vi "PPS Close.vi"(8 "error in (no error)":errorcluster, 11 "IT-M3904D in":refnum<class "IT-M3904D.lvclass">) -> (0 "error out":errorcluster, 3 "IT-M3904D out":refnum<class "IT-M3904D.lvclass">)   [LabVIEW 2023, in "HardwareAbstractionLayer_LVOOP.lvlib" / "IT-M3904D.lvclass"]
uses:
  IT-M3904D.lvclass
  <instrlib>/IT-M3900D/IT-M3900D.lvlib
  PowerSupply.lvclass
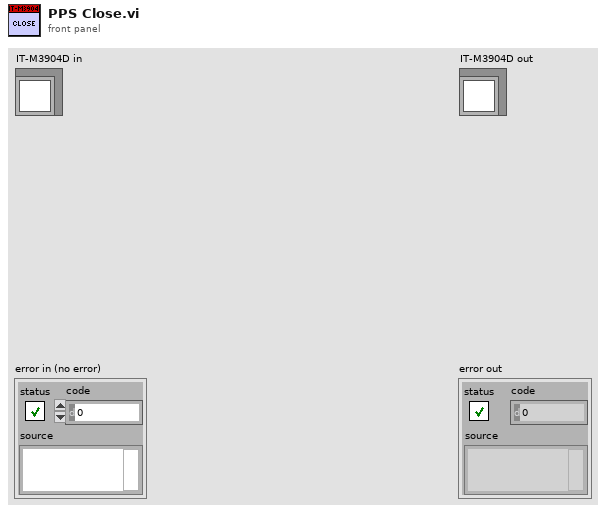
[diagram p1: front panel]
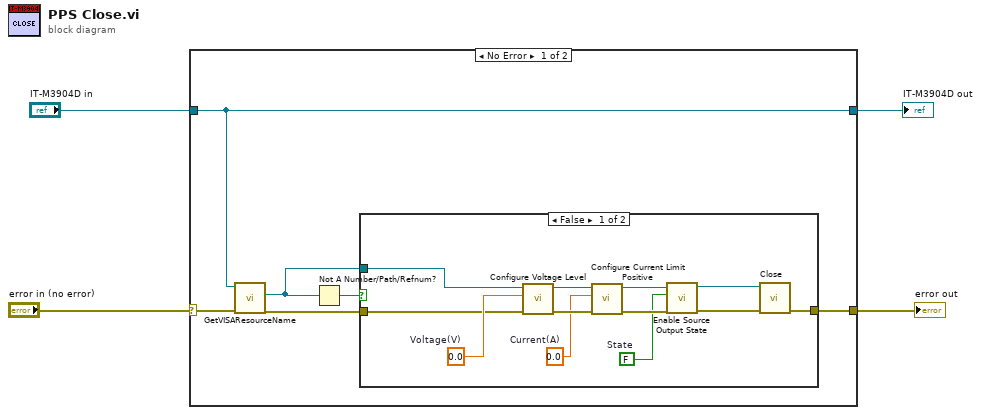
[diagram p0: block diagram]
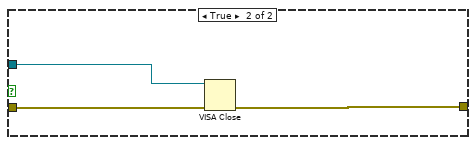
[diagram p2: hidden frame]
diagram:
  n1 = case shown="No Error" "error in (no error)" {
    selector: "error in (no error)" -> [w9 w26]
    tunnel: [w10 w26] -> w3
    tunnel: "IT-M3904D in" -> [w8 w27]
    tunnel: [w8 w27] -> w1
    frame No Error {
      n2 = call "GetVISAResourceName.vi"("error in (no error)"=w9, "object in"=w8) -> ("error out"=w7:errorcluster, "VISA resource name"=w6:refnum<visa-resource-name>)  [unwired: 7 in, 1 out]
      n3 = Not A Number/Path/Refnum?(number/path/refnum=w6) -> (NaN/Path/Refnum?=w5:bool)
      n4 = case shown="False" w5 {
        tunnel: [w22 w24] -> w10
        tunnel: w7 -> [w14 w25]
        tunnel: w6 -> [w11 w23]
        frame False {
          w15 = FALSE  # State
          w16 = 0.0  # Current(A)
          w17 = 0.0  # Voltage(V)
          n5 = call <instrlib>:"Configure Voltage Level.vi"("error in"=w14, "Voltage(V)"=w17, "VISA resource name"=w11) -> ("error out"=w20:errorcluster, "VISA resource name out"=w21:refnum<visa-resource-name>)  [unwired: 7 in]
          n6 = call <instrlib>:"Configure Current Limit Positive.vi"("error in"=w20, "Value(A)"=w16, "VISA resource name"=w21) -> ("error out"=w18:errorcluster, "VISA resource name out"=w19:refnum<visa-resource-name>)  [unwired: 7 in]
          n7 = call <instrlib>:"Enable Source Output State.vi"("error in"=w18, "State"=w15, "VISA resource name"=w19) -> ("error out"=w13:errorcluster, "VISA resource name out"=w12:refnum<visa-resource-name>)  [unwired: 7 in]
          n8 = call <instrlib>:"Close.vi"("error in"=w13, "VISA resource name"=w12) -> ("error out"=w22:errorcluster)  [unwired: 9 in]
        }
        frame True {
          n9 = VISA Close(VISA resource name=w23, error in (no error)=w25) -> (error out=w24:errorcluster)
        }
      }
    }
    frame Error {
    }
  }
  "error out" <- w3
  "IT-M3904D out" <- w1
